vi "Close Instrument.vi"(8 "error in (no error)":errorcluster, 11 "Instrument.VRM in":refnum<class "Instrument.OxfordVRM.lvclass">) -> (0 "error out":errorcluster, 3 "Instrument.VRM out":refnum<class "Instrument.OxfordVRM.lvclass">)   [LabVIEW 2016, in "Instrument.OxfordVRM.lvclass"]
uses:
  Instrument.OxfordVRM.lvclass
  <instrlib>/Mercury iXX/Public/Controls/Mercury Reference.ctl
  <instrlib>/Mercury iXX/Public/Controls/Comms Transport Layer.ctl
  <instrlib>/Mercury iXX/Private/Controls/Query Dynamic Reference.ctl
  Instrument.OxfordVRM.lvclass/Instrument.OxfordVRM.ctl
  <instrlib>/Mercury iXX/Mercury iXX.lvlib
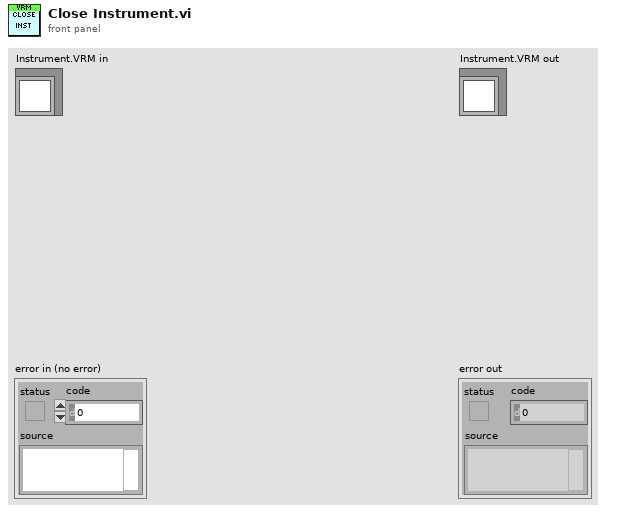
[diagram p1: front panel]
types:
  T1 = typedef "Mercury iXX.lvlib/Mercury Reference.ctl" = cluster{"Comms":refnum<visa-resource-name>, "Device ID":string[], "Comms Layer":T2, "Command":string, "Query reference":T3}
  T2 = typedef "Mercury iXX.lvlib/Comms Transport Layer.ctl" = enum16{"Ethernet TCP/IP", "USB", "ISOBus - RS-232", "GPIB"}
  T3 = typedef "Mercury iXX.lvlib/Query Dynamic Reference.ctl" = refnum<vi>
  T4 = cluster{"Address":string, "Reference":T1, "Devices":cluster{"Temperature":string, "Magnet X":string, "Magnet Y":string, "Magnet Z":string, "PSU 1":string, "PSU 2":string, "PSU 3":string, "PSU 4":string, "PSU 5":string, "PSU 6":string}}
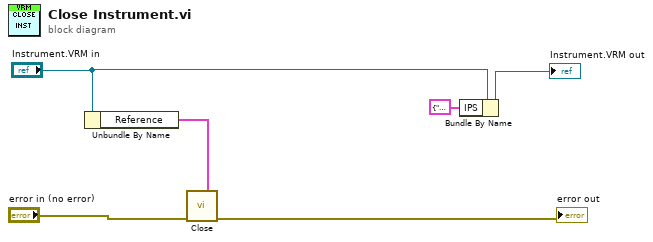
[diagram p0: block diagram]
diagram:
  n1 = Unbundle By Name("Instrument.VRM in") -> ("Reference"=w4:T1)
  n2 = call <instrlib>:"Close.vi"("error in (no error)"="error in (no error)", "Mercury Reference"=w4) -> ("error out"=→"error out":errorcluster)  [unwired: 9 out]
  n3 = Bundle By Name(cluster="Instrument.VRM in", "IPS"=T4 {"Address"="", "Reference"={"Comms"="", "Device ID"=[], "Comms Layer"=enum."Ethernet TCP/IP", "Command"="", "Query reference"=refnum}, "Devices"={"Temperature"="", "Magnet X"="", "Magnet Y"="", "Magnet Z"="", "PSU 1"="", "PSU 2"="", "PSU 3"="", "PSU 4"="", "PSU 5"="", "PSU 6"=""}}) -> (→"Instrument.VRM out":refnum<class "Instrument.OxfordVRM.lvclass">)
